vi "create Renderer With Time Shift And Channels.vi"(0 "pRendererId":i32, 1 "pMaxTextureWidth":i32, 2 "pTimeShift":bool, 5 "pWindowWidth":i32, 7 "pWindowHeight":i32, 9 "pBytesPerVoxel":i32, 11 "error in (no error)":errorcluster, 12 "pMaxTextureHeight":i32, 13 "pChannelSelector":bool) -> (4 "function return":i32, 15 "error out":errorcluster)   [LabVIEW 2012, in "clearvolume.lvlib"]
doc: "__declspec(dllexport) long __cdecl createRendererWithTimeShiftAndChannels( long pRendererId,\n long pWindowWidth,\n long pWindowHeight,\n long pBytesPerVoxel,\n long pMaxTextureWidth,\n long pMaxTextureHeight,\n bool pTimeShift,\n bool pChannelSelector);"
uses:
  clearvolume.lvlib
  clearvolume.dll
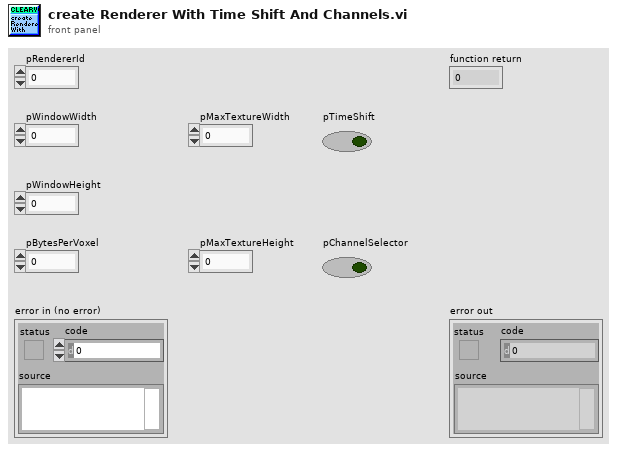
[diagram p1: front panel]
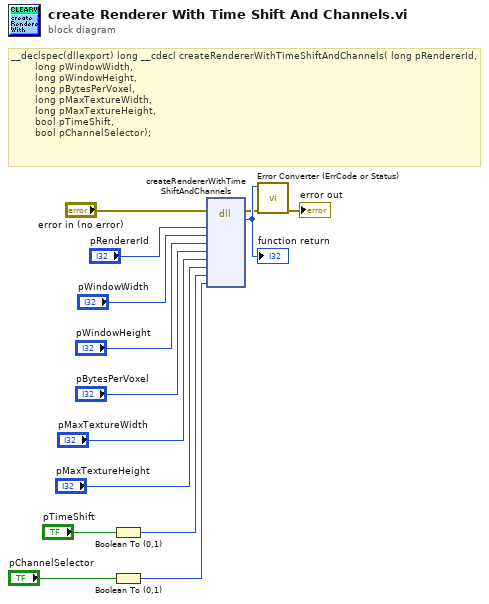
[diagram p0: block diagram]
diagram:
  # "__declspec(dllexport) long __cdecl createRendererWithTimeShiftAndChannels(\tlong pRendererId,\n        long pWindowWidth,\n        long pWindowHeight,\n        long pBytesPerVoxel,\n        long pMaxTextureWidth,\n        long pMaxTextureHeight,\n        bool pTimeShift,\n        bool pChannelSelector);"
  n1 = Boolean To (0,1)(Boolean="pTimeShift") -> (0, 1=w6:i16)
  n2 = Boolean To (0,1)(Boolean="pChannelSelector") -> (0, 1=w4:i16)
  n3 = dll-call lib="C:/Users/myerslab/workspace/Libraries/CV/clearvolume/src/labview/clearvolume/clearvolume.*" fn="createRendererWithTimeShiftAndChannels"(error in="error in (no error)", "pRendererId"="pRendererId", "pWindowWidth"="pWindowWidth", "pWindowHeight"="pWindowHeight", "pBytesPerVoxel"="pBytesPerVoxel", "pMaxTextureWidth"="pMaxTextureWidth", "pMaxTextureHeight"="pMaxTextureHeight", "pTimeShift"=w6, "pChannelSelector"=w4) -> (error out=w2:errorcluster, w14:i32)  [unwired: 10 in, 1 out]
  "function return" <- w14
  n4 = call "Error Converter (ErrCode or Status).vi"("error in (no error)"=w2, "error code"=w14) -> ("error out"=→"error out":errorcluster)  [unwired: 9 in]
